vi "test Disable Enable Routing Channel.vi"(8 "error in (no error)":errorcluster, 11 "TestCase in":refnum<class "Routing and Faulting Scripting Unit Tests.lvclass">) -> (0 "error out":errorcluster, 3 "TestCase out":refnum<class "Routing and Faulting Scripting Unit Tests.lvclass">)   [LabVIEW 2020, in "Routing and Faulting Scripting Unit Tests.lvclass"]
uses:
  Routing and Faulting Scripting Unit Tests.lvclass
  Routing and Faulting Scripting Unit Tests.lvclass/Routing and Faulting Scripting Unit Tests.ctl
  NationalInstruments.VeriStand.SystemDefinitionAPI
  <vilib>/addons/_JKI Toolkits/VI Tester/TestCase.llb/TestCase.lvclass
  Routing and Faulting Scripting.lvlib
  C:/Program Files (x86)/National Instruments/LabVIEW 2020/vi.lib/addons/_JKI Toolkits/VI Tester/TestCase.llb/TestCase.lvclass
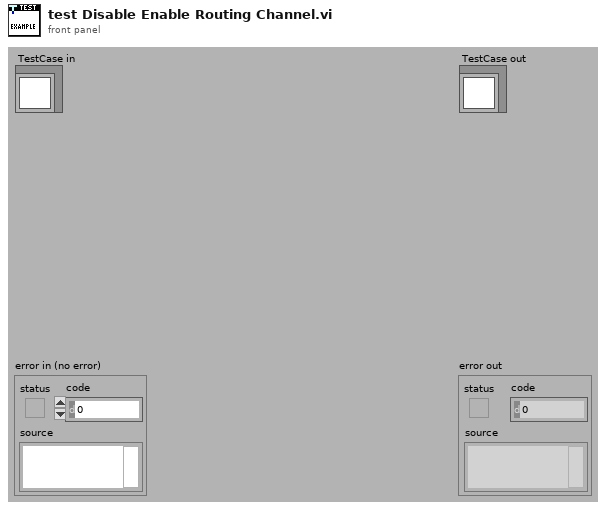
[diagram p1: front panel]
types:
  T1 = typedef "Custom Device API.lvlib/Custom Device Item Ref.ctl" = u64
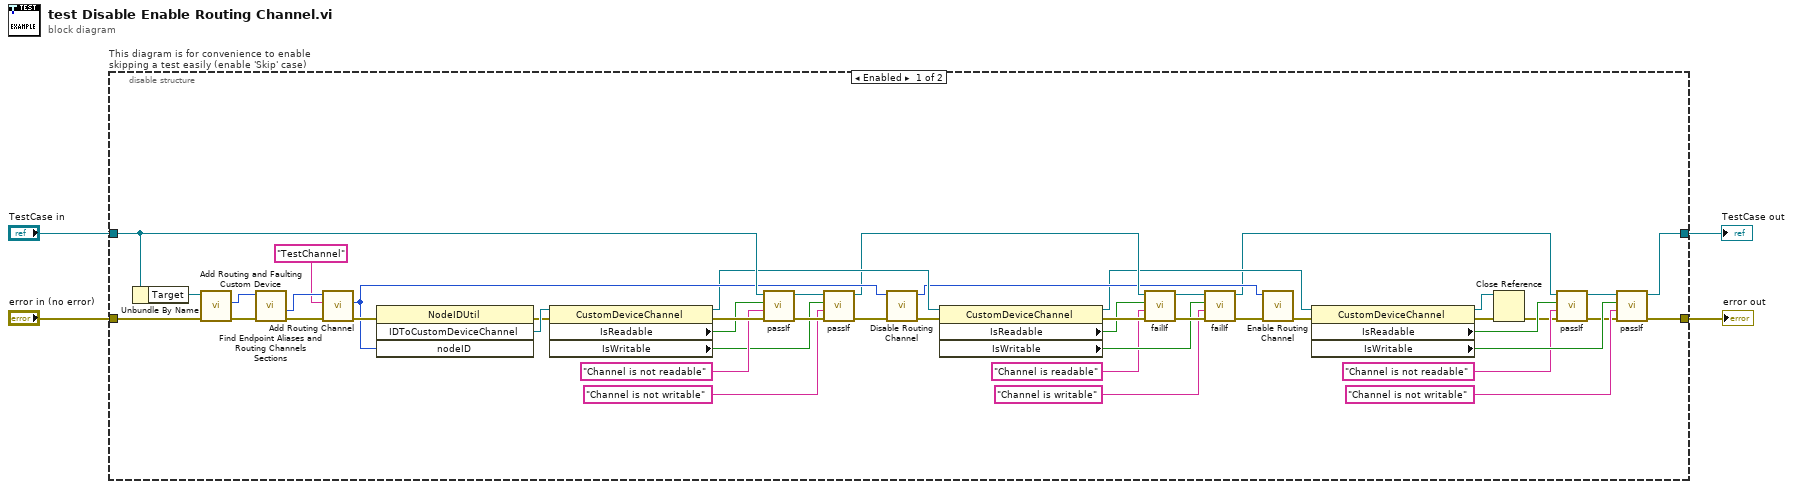
[diagram p0: block diagram]
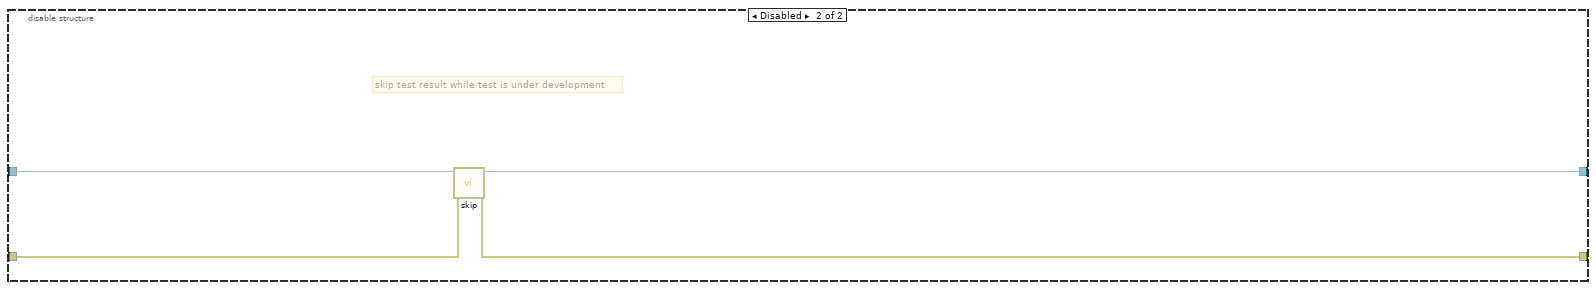
[diagram p2: hidden frame]
diagram:
  n1 = disable-structure "This diagram is for convenience to enable skipping a test easily (enable 'Skip' case)" shown="Enabled" {
    disable-tunnel: "TestCase in" -> [w38 w54]
    disable-tunnel: [w7 w52] -> w1
    disable-tunnel: [w41 w53] -> w3
    disable-tunnel: "error in (no error)" -> [w50 w51]
    frame Enabled {
      n2 = Unbundle By Name(w38) -> ("Target"=w49:refnum<k24>)
      n3 = call "Add Routing and Faulting Custom Device.vi"("error in"=w50, "target in"=w49) -> ("error out"=w48:errorcluster, "routing and faulting custom device"=w47:T1)  [unwired: 7 in, 1 out]
      n4 = call "Find Endpoint Aliases and Routing Channels Sections.vi"("error in"=w48, "routing and faulting custom device in"=w47) -> ("error out"=w46:errorcluster, "routing channels"=w45:T1)  [unwired: 6 in, 2 out]
      n5 = call "Add Routing Channel.vi"("error in"=w46, "channel name"="TestChannel" ("Channel Name"), "routing channels in"=w45) -> ("error out"=w43:errorcluster, "routing channel"=w30:T1)  [unwired: 6 in, 1 out]
      n6 = invoke class="NodeIDUtil" method="IDToCustomDeviceChannel"(error in=w43, "nodeID"=w30) -> (error out=w40:errorcluster, "IDToCustomDeviceChannel"=w42:refnum<k24>)  [unwired: 2 in, 2 out]
      n7 = property class="CustomDeviceChannel"(reference=w42, error in=w40) -> (reference out=w28:refnum<k24>, error out=w39:errorcluster, "IsReadable"=w37:bool, "IsWritable"=w33:bool)
      n8 = call-dynamic "passIf.vi"("error in (no error)"=w39, "message (\"\")"="Channel is not readable" ("message (\"\")"), "pass"=w37, "TestCase in"=w38) -> ("error out"=w34:errorcluster, "TestCase out"=w35:refnum<class "Routing and Faulting Scripting Unit Tests.lvclass">)  [unwired: 6 in]
      n9 = call-dynamic "passIf.vi"("error in (no error)"=w34, "message (\"\")"="Channel is not writable" ("message (\"\")"), "pass"=w33, "TestCase in"=w35) -> ("error out"=w31:errorcluster, "TestCase out"=w25:refnum<class "Routing and Faulting Scripting Unit Tests.lvclass">)  [unwired: 6 in]
      n10 = call "Disable Routing Channel.vi"("error in"=w31, "routing channel in"=w30) -> ("error out"=w29:errorcluster, "routing channel out"=w18:T1)  [unwired: 8 in]
      n11 = property class="CustomDeviceChannel"(reference=w28, error in=w29) -> (reference out=w9:refnum<k24>, error out=w27:errorcluster, "IsReadable"=w24:bool, "IsWritable"=w22:bool)
      n12 = call-dynamic "failIf.vi"("error in (no error)"=w27, "message (\"\")"="Channel is readable" ("message (\"\")"), "fail"=w24, "TestCase in"=w25) -> ("error out"=w23:errorcluster, "TestCase out"=w26:refnum<class "Routing and Faulting Scripting Unit Tests.lvclass">)  [unwired: 6 in]
      n13 = call-dynamic "failIf.vi"("error in (no error)"=w23, "message (\"\")"="Channel is writable" ("message (\"\")"), "fail"=w22, "TestCase in"=w26) -> ("error out"=w19:errorcluster, "TestCase out"=w8:refnum<class "Routing and Faulting Scripting Unit Tests.lvclass">)  [unwired: 6 in]
      n14 = call "Enable Routing Channel.vi"("error in"=w19, "routing channel in"=w18) -> ("error out"=w10:errorcluster)  [unwired: 8 in, 1 out]
      n15 = property class="CustomDeviceChannel"(reference=w9, error in=w10) -> (reference out=w5:refnum<k24>, error out=w11:errorcluster, "IsReadable"=w12:bool, "IsWritable"=w16:bool)
      n16 = Close Reference(reference=w5, error in (no error)=w11) -> (error out=w6:errorcluster)
      n17 = call-dynamic "passIf.vi"("error in (no error)"=w6, "message (\"\")"="Channel is not readable" ("message (\"\")"), "pass"=w12, "TestCase in"=w8) -> ("error out"=w15:errorcluster, "TestCase out"=w14:refnum<class "Routing and Faulting Scripting Unit Tests.lvclass">)  [unwired: 6 in]
      n18 = call-dynamic "passIf.vi"("error in (no error)"=w15, "message (\"\")"="Channel is not writable" ("message (\"\")"), "pass"=w16, "TestCase in"=w14) -> ("error out"=w41:errorcluster, "TestCase out"=w7:refnum<class "Routing and Faulting Scripting Unit Tests.lvclass">)  [unwired: 6 in]
    }
    frame Disabled {
      # "skip test result while test is under development"
      n19 = call <vilib>:"skip.vi"("error in (no error)"=w51, "TestCase in"=w54) -> ("error out"=w53:errorcluster, "TestCase out"=w52:refnum<class "Routing and Faulting Scripting Unit Tests.lvclass">)  [unwired: 8 in]
    }
  }
  "error out" <- w3
  "TestCase out" <- w1
